vi "robot tracker2.vi"(4 "initialize":bool, 5 "speeds":cluster{"right speed":dbl, "left speed":dbl} {"left speed" step=0.05000000074505806 scale=-1.0..1.0; "right speed" step=0.05000000074505806 scale=-1.0..1.0}, 7 "configuration":T2={"default picture"=bytes[0], "default direction"=0.0, "pixel width between wheels"=20.0, "initial robot location"={"x"=0, "y"=0}, "R color"=6618880, "L color"=16711680}) -> (1 "feedback":T1={"left coord"={"x"=300.0, "y"=600.0}, "right coord"={"x"=310.0, "y"=600.0}, "direction indicator"=0.0, "robot location"={"x"=0.0, "y"=0.0}} {"direction indicator" scale=0.0..6.28323}, 3 "Picture":picture)   [LabVIEW 2009]
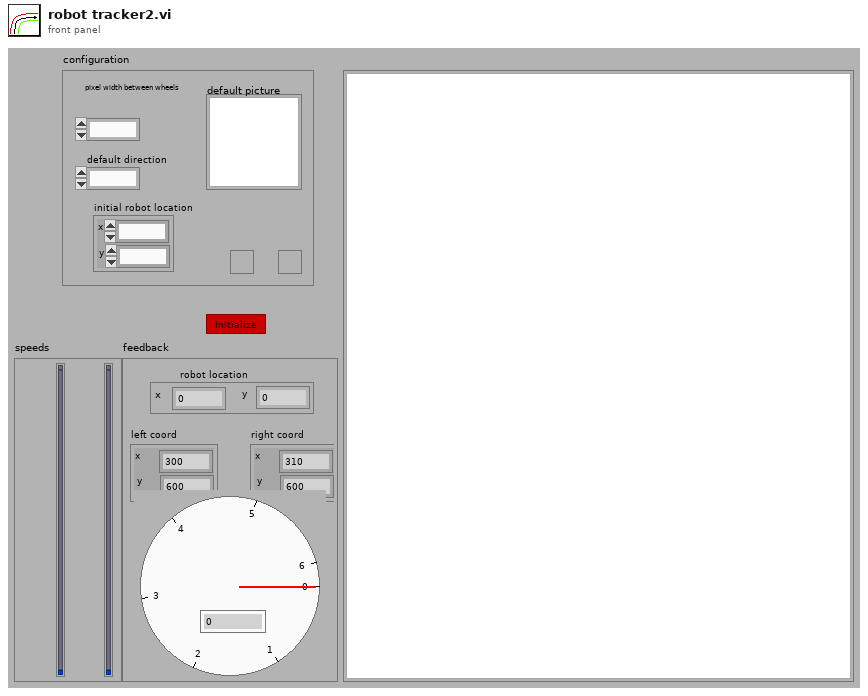
[diagram p1: front panel]
types:
  T1 = cluster{"left coord":cluster{"x":dbl, "y":dbl}, "right coord":cluster{"x":dbl, "y":dbl}, "direction indicator":sgl, "robot location":cluster{"x":dbl, "y":dbl}}
  T2 = cluster{"default picture":picture, "default direction":sgl, "pixel width between wheels":dbl, "initial robot location":cluster{"x":i16, "y":i16}, "R color":u32, "L color":u32}
  T3 = cluster{cluster{dbl, dbl}, cluster{dbl, dbl}, "default direction":sgl, "initial robot location":cluster{"x":i16, "y":i16}}
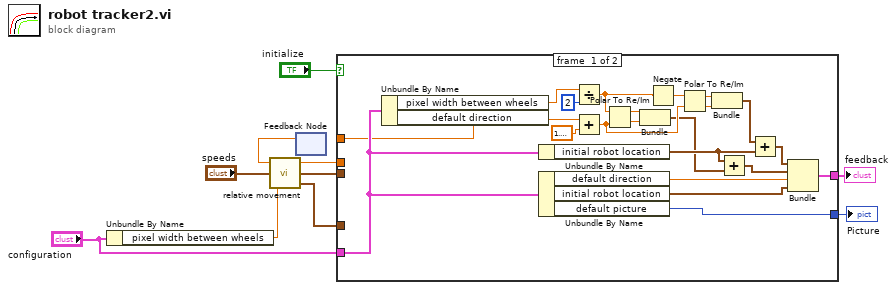
[diagram p0: block diagram]
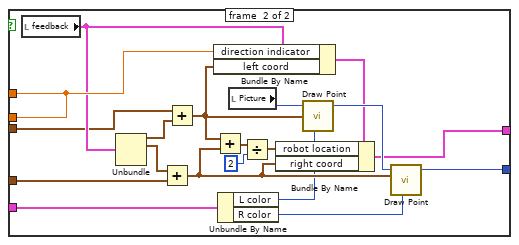
[diagram p2: hidden frame]
diagram:
  n1 = Unbundle By Name("configuration") -> ("pixel width between wheels"=w5:dbl)
  n2 = feedback #1() -> (w10:dbl)  [unwired: 1 in]
  n3 = call "relative movement.vi"("representative width between wheels"=w5, "speeds"="speeds", "start direction"=w10) -> ("right position"=w1:cluster{dbl, dbl}, "left position"=w2:cluster{dbl, dbl}, "direction"=w3:dbl)
  n4 = case shown="True" "initialize" {
    tunnel: [w32 w45] -> w11
    tunnel: [w17 w37] -> w9
    tunnel: w3 -> [_ w37]
    tunnel: [w18 w36] -> w7
    tunnel: "configuration" -> [w21 w40]
    tunnel: w2 -> [_ w34]
    tunnel: w1 -> [_ w33]
    frame #0 {
      n5 = Unbundle By Name(w21) -> ("pixel width between wheels"=w30:dbl, "default direction"=w17:sgl)
      n6 = Unbundle By Name(w21) -> ("initial robot location"=w14:cluster{"x":i16, "y":i16})
      n7 = Unbundle By Name(w21) -> ("default direction"=w15:sgl, "initial robot location"=w19:cluster{"x":i16, "y":i16}, "default picture"=w32:picture)
      n8 = Divide(x=w30, y=2) -> (x/y=w26:dbl)
      n9 = Add(x=w17, y=1.5707963267948966) -> (x+y=w28:dbl)
      n10 = Polar To Re/Im(2:w28, 3:w26) -> (0:w24:dbl, 1:w25:dbl)
      n11 = Bundle(w25, w24) -> (w13:cluster{dbl, dbl})  [unwired: 1 in]
      n12 = Negate(x=w26) -> (-x=w27:dbl)
      n13 = Polar To Re/Im(2:w28, 3:w27) -> (0:w23:dbl, 1:w22:dbl)
      n14 = Bundle(w22, w23) -> (w20:cluster{dbl, dbl})  [unwired: 1 in]
      n15 = Add(x=w14, y=w13) -> (x+y=w12:cluster{dbl, dbl})
      n16 = Add(x=w20, y=w14) -> (x+y=w16:cluster{dbl, dbl})
      n17 = Bundle(w16, w12, "default direction"=w15, "initial robot location"=w19) -> (w18:T3)  [unwired: 1 in]
    }
    frame #1 {
      n18 = local read "feedback"() -> (w35:T1)
      n19 = Unbundle(w35) -> ("left coord"=w47:cluster{"x":dbl, "y":dbl}, "right coord"=w48:cluster{"x":dbl, "y":dbl})  [unwired: 2 out]
      n20 = Add(x=w48, y=w33) -> (x+y=w41:cluster{dbl, dbl})
      n21 = Add(x=w34, y=w47) -> (x+y=w46:cluster{dbl, dbl})
      n22 = Bundle By Name(cluster=w35, "direction indicator"=w37, "left coord"=w46) -> (w43:T1)
      n23 = Add(x=w46, y=w41) -> (x+y=w51:cluster{dbl, dbl})
      n24 = Unbundle By Name(w40) -> ("L color"=w39:u32, "R color"=w38:u32)
      n25 = local read "Picture"() -> (w50:picture)
      n26 = Divide(x=w51, y=2) -> (x/y=w42:cluster{dbl, dbl})
      n27 = Bundle By Name(cluster=w43, "robot location"=w42, "right coord"=w41) -> (w36:T1)
      n28 = call <vilib>:"Draw Point.vi"("picture"=w50, "point(x,y)"=w46, "color(black)"=w39) -> ("new picture"=w49:picture)  [unwired: 6 in]
      n29 = call <vilib>:"Draw Point.vi"("picture"=w49, "point(x,y)"=w41, "color(black)"=w38) -> ("new picture"=w45:picture)  [unwired: 6 in]
    }
  }
  "Picture" <- w11
  "feedback" <- w7
